vi "libtiff2_close.vi"(7 "error in (no error)":errorcluster, 10 "Handle":i32) -> (0 "error out":errorcluster)   [LabVIEW 2012]
doc: "Close a file open for reading or writing"
uses:
  C:/Program Files (x86)/GnuWin32/bin/libtiff3.dll
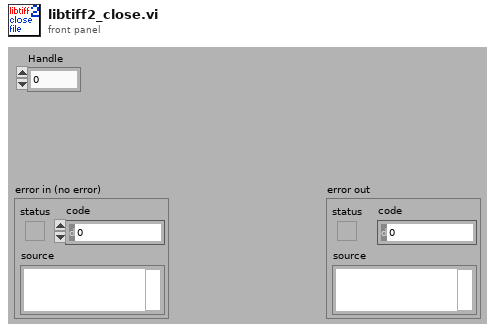
[diagram p1: front panel]
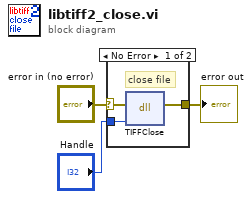
[diagram p0: block diagram]
diagram:
  n1 = case shown="No Error" "error in (no error)" {
    selector: "error in (no error)" -> [w4 w7]
    tunnel: "Handle" -> [w6 _]
    tunnel: [w5 w7] -> w2
    frame No Error {
      # "close file"
      n2 = dll-call lib="C:/Program Files (x86)/GnuWin32/bin/libtiff3.dll" fn="TIFFClose"(error in=w4, "Handle"=w6) -> (error out=w5:errorcluster)  [unwired: 3 in, 2 out]
    }
    frame Error {
    }
  }
  "error out" <- w2
